vi "Set Inline Buffer.vi"(8 "error in (no error)":errorcluster, 10 "command parameters":T1, 11 "Plugin Thread in":refnum<class "Plugin Thread.lvclass">) -> (0 "error out":errorcluster, 3 "Plugin Thread out":refnum<class "Plugin Thread.lvclass">)   [LabVIEW 2019, in "DSF Core.lvlib" / "Plugin Thread.lvclass"]
uses:
  Thread/Plugin/Plugin Thread.lvclass
  Interface/Plugin/Command Parameters.ctl
  Buffer/Buffer.lvclass
  C:/Program Files (x86)/National Instruments/LabVIEW 2019/vi.lib/NI/Memory Manager/Classes/Pointer/Pointer.lvclass
  <vilib>/NI/Memory Manager/Classes/Pointer/Pointer.lvclass/Pointer.ctl
  Thread/Plugin/Plugin Thread.lvclass/Plugin Thread.ctl
  <vilib>/NI/Memory Manager/Classes/Pointer/Set Size.vi
  <vilib>/NI/Memory Manager/Classes/Pointer/Set Address.vi
  <vilib>/NI/Memory Manager/Classes/Pointer/Check Null Pointer.vi
  <vilib>/NI/Memory Manager/Classes/Pointer/Set Internal.vi
  <vilib>/NI/Memory Manager/Classes/Pointer/Errors.vi
  <vilib>/NI/Memory Manager/Classes/Pointer/Null Pointer.vi
  <vilib>/NI/Memory Manager/Classes/Pointer/Is Null.vi
  <vilib>/NI/Memory Manager/Classes/Pointer/Create Error.vi
  <vilib>/NI/Memory Manager/Classes/Pointer/Get Address.vi
  <vilib>/NI/Memory Manager/VIs/New Error Cluster.vi
  <vilib>/NI/Memory Manager/VIs/New Error Cluster (512B).vi
  <vilib>/NI/Memory Manager/VIs/Set Error Status.vi
  <vilib>/NI/Memory Manager/VIs/Set Error Code.vi
  <vilib>/NI/Memory Manager/VIs/Set Error Source.vi
  <vilib>/NI/Memory Manager/Constants/Constants.vi
  <vilib>/NI/Memory Manager/Constants/Library Name.vi
  <vilib>/NI/Memory Manager/Classes/Pointer/Pointer Error Info.vi
  <vilib>/NI/Memory Manager/VIs/Write String to Source.vi
  <vilib>/NI/Memory Manager/Constants/Pointer Class Name.vi
  <vilib>/NI/Memory Manager/Classes/Pointer/Pointer.lvclass
  Transfer Group/Transfer Group.lvclass
  Interface/Plugin/Plugin Interface.lvclass
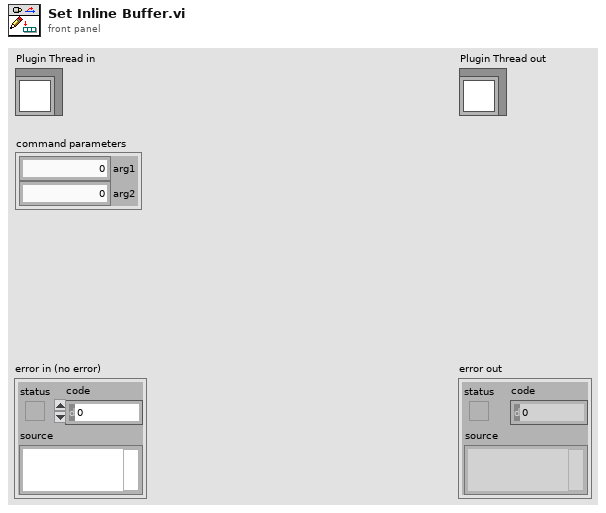
[diagram p1: front panel]
types:
  T1 = typedef "DSF Core.lvlib/Plugin Interface.lvclass/Command Parameters.ctl" = cluster{"arg1":u64, "arg2":u64}
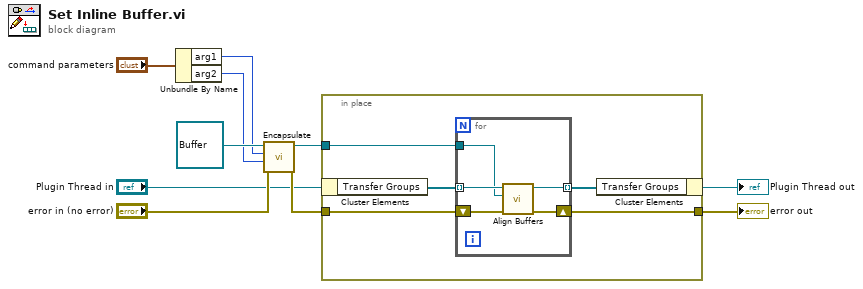
[diagram p0: block diagram]
diagram:
  n1 = Unbundle By Name("command parameters") -> ("arg1"=w6:u64, "arg2"=w7:u64)
  n2 = call <vilib>:"Encapsulate.vi"("error in (no error)"="error in (no error)", "size"=w7, "address"=w6, "Pointer type"=refnum<class "Buffer.lvclass"> refnum ("base Buffer")) -> ("error out"=w3:errorcluster, "Pointer"=w2:refnum<class "Buffer.lvclass">)  [unwired: 6 in]
  n3 = in-place {
    in-place-border: [w14] -> w4
    in-place-border: w3 -> [w12]
    in-place-border: w2 -> [w11]
    n4 = in-place-cluster #1("Plugin Thread in") -> ("Transfer Groups"=w13:refnum<class "Transfer Group.lvclass">[])
    n5 = for {
      tunnel: w13 -> [w20] mode=indexing
      tunnel: [w19] -> w15 mode=indexing
      shift-right: [w18] -> w14
      shift-left: w12 -> [w17]
      tunnel: w11 -> [w16]
      n6 = call "Align Buffers.vi"("error in (no error)"=w17, "base Inline Buffer"=w16, "Transfer Group in"=w20) -> ("error out"=w18:errorcluster, "Transfer Group out"=w19:refnum<class "Transfer Group.lvclass">)  [unwired: 7 in]
    }
    n7 = in-place-cluster #1("Transfer Groups"=w15) -> (→"Plugin Thread out":refnum<class "Plugin Thread.lvclass">)
  }
  "error out" <- w4
